vi "To Byte Array (U16).vi"(1 "element in":u16) -> (0 "byte array out":u8[](array[numeric]) format="%x")   [LabVIEW 2013]
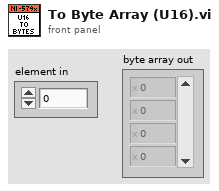
[diagram p1: front panel]
types:
  T1 = enum16{"big-endian, network order", "native, host order", "little-endian"}
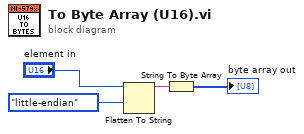
[diagram p0: block diagram]
diagram:
  n1 = Flatten To String(anything="element in", byte order (0:big-endian, network order)=T1."little-endian") -> (data string=w3:string)  [unwired: 2 in, 2 out]
  n2 = String To Byte Array(string=w3) -> (unsigned byte array=→"byte array out":u8[])
